vi "Table-Check valid column selected.vi"(8 "error in (no error)":errorcluster, 9 "Cell Position":T1, 11 "Table ref in":refnum<vi>) -> (0 "error out":errorcluster, 1 "Selected cell":cluster{"Sel Row":i32, "Sel Column":i32}, 2 "Selected cell validity cluster":T2, 3 "Table ref":refnum<vi>, 4 "Edit Position":T3)   [LabVIEW 2020]
uses:
  <vilib>/Utility/miscctls.llb/LVRowAndColumnTypeDef.ctl
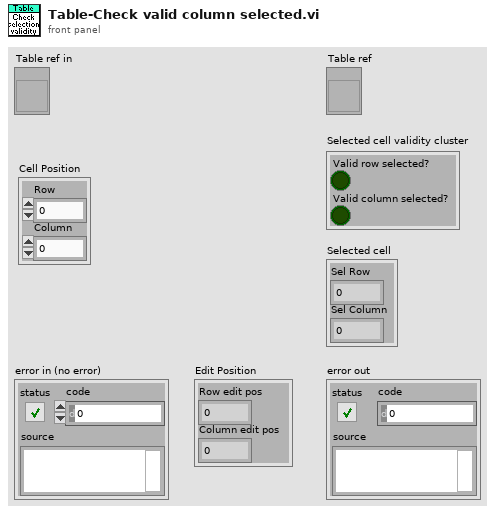
[diagram p1: front panel]
types:
  T1 = typedef "LVRowAndColumnTypeDef.ctl" = cluster{"Row":i32, "Column":i32}
  T2 = cluster{"Valid row selected?":bool, "Valid column selected?":bool}
  T3 = cluster{"Row edit pos":i32, "Column edit pos":i32}
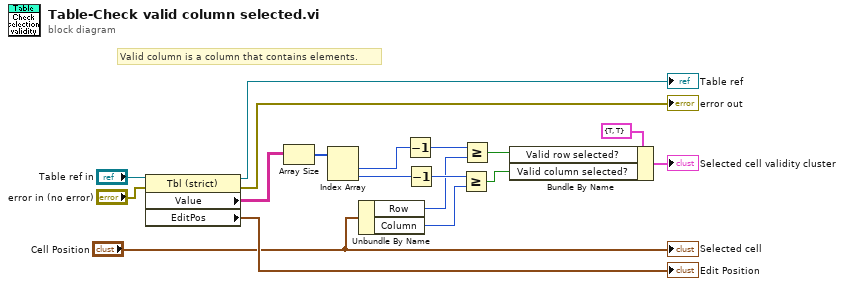
[diagram p0: block diagram]
diagram:
  # "Valid column is a column that contains elements."
  n1 = property on="Property Node" class="Tbl (strict)"(reference="Table ref in", error in="error in (no error)") -> (reference out=→"Table ref":refnum<vi>, error out=→"error out":errorcluster, "Value"=w17:string[][], "EditPos"=→"Edit Position":T1)
  n2 = Array Size(array=w17) -> (size(s)=w12:i32[])
  n3 = Index Array(array=w12) -> (element #1=w7:i32, element #2=w13:i32)  [unwired: 2 in]
  n4 = Unbundle By Name("Cell Position") -> ("Row"=w2:i32, "Column"=w11:i32)
  n5 = Decrement(x=w7) -> (x-1=w8:i32)
  n6 = Decrement(x=w13) -> (x-1=w14:i32)
  n7 = Greater Or Equal?(x=w14, y=w11) -> (x >= y?=w3:bool)
  n8 = Greater Or Equal?(x=w8, y=w2) -> (x >= y?=w4:bool)
  n9 = Bundle By Name(cluster=T2 {"Valid row selected?"=TRUE, "Valid column selected?"=TRUE} ("Validity cluster"), "Valid row selected?"=w4, "Valid column selected?"=w3) -> (→"Selected cell validity cluster":T2)
  "Selected cell" <- "Cell Position"
